vi "reaction_quantity.vi"(9 "angle_input":i16, 10 "gravitational_constant":dbl, 11 "mass":dbl) -> (3 "reaction":dbl)   [LabVIEW 2018]
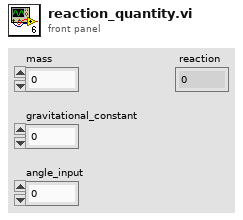
[diagram p1: front panel]
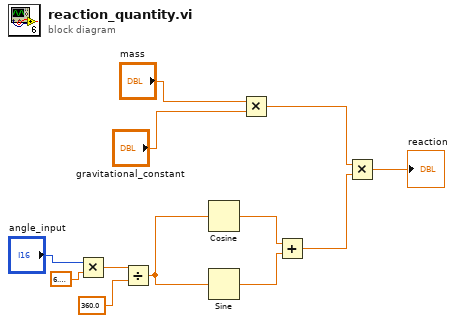
[diagram p0: block diagram]
diagram:
  n1 = Multiply(x="angle_input", y=6.283185307179586) -> (x*y=w3:dbl)
  n2 = Divide(x=w3, y=360.0) -> (x/y=w1:dbl)
  n3 = Cosine(x=w1) -> (cos(x)=w6:dbl)
  n4 = Sine(x=w1) -> (sin(x)=w7:dbl)
  n5 = Multiply(x="mass", y="gravitational_constant") -> (x*y=w11:dbl)
  n6 = Add(x=w6, y=w7) -> (x+y=w10:dbl)
  n7 = Multiply(x=w11, y=w10) -> (x*y=→"reaction":dbl)
